vi "Test Encode to File Buffer.vi"(8 "error in (no error)":errorcluster, 11 "01_Image in":refnum<class "01_Image.lvclass">) -> (0 "error out":errorcluster, 3 "01_Image out":refnum<class "01_Image.lvclass">)   [LabVIEW 2020, in "test.lvlib" / "01_Image.lvclass"]
uses:
  01_Image.lvclass
  C:/Program Files (x86)/National Instruments/LabVIEW 2020/vi.lib/Astemes/LUnit/Test Case.lvclass
  common/Image Size (Integer).ctl
  <vilib>/Astemes/LUnit/Test Case.lvclass/Test Case.ctl
  image/Image to File-Buffer Encoder/Image to File-Buffer Encoder.lvclass/Image to File-Buffer Encoder.ctl
  21d28007-5dca-4d87-b59f-e9153fb71e50.vi
  image/Image to File-Buffer Encoder/Encode Image (ARGB).vi
  fadc1fe5-6c10-4d26-80da-2e71b1445ac9.vi
  image/New Image.vi
  image/New Image (ARGB Preallocated).vi
  image/Copy Array to Image.vi
  image/Copy Array to Image (ARGB).vi
  image/Encode Image to File Buffer (ARGB).vi/b711c62e-7e14-408f-bb3b-a3086b0dc120.vi
  <vilib>/Astemes/LUnit/Core/LUnit Test Case/Private/Append Pass Result.vi
  <vilib>/Astemes/LUnit/Core/LUnit Test Case/Private/Append Fail Result.vi
  21d28007-5dca-4d87-b59f-e9153fb71e50.vi/9c5d11cd-9439-4240-a1ee-d9baace9c924.vi
  image/Image to File-Buffer Encoder/Encode Image (ARGB).vi/c8136873-c742-4257-b221-98e07a73ef51.vi
  fadc1fe5-6c10-4d26-80da-2e71b1445ac9.vi/9c5d11cd-9439-4240-a1ee-d9baace9c924.vi
  image/New Image (ARGB Preallocated).vi/3321fa97-f432-4e1e-8db9-a0df79aed21b.vi
  image/ARGB Colour to U32 Pixel Value.vi
  <vilib>/Astemes/LUnit/Core/LUnit Test Case/Private/Run In UI.vi
  <vilib>/Utility/error.llb/Clear Errors.vi
  <vilib>/Utility/error.llb/Error Cluster From Error Code.vi
  <vilib>/picture/pixmap.llb/Flatten Pixmap.vi
  image/Image to File-Buffer Encoder/Create (with Extension).vi
  common/common.lvlib
  image/image.lvlib
  image/Image to File-Buffer Encoder/Image to File-Buffer Encoder.lvclass
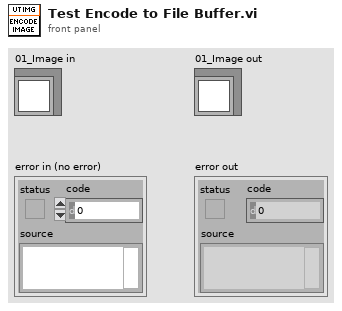
[diagram p1: front panel]
types:
  T1 = typedef "common.lvlib/Image Size (Integer).ctl" = cluster{"Width":u16, "Height":u16}
  T2 = typedef "image.lvlib/ARGB Image.ctl" = refnum<data-value>
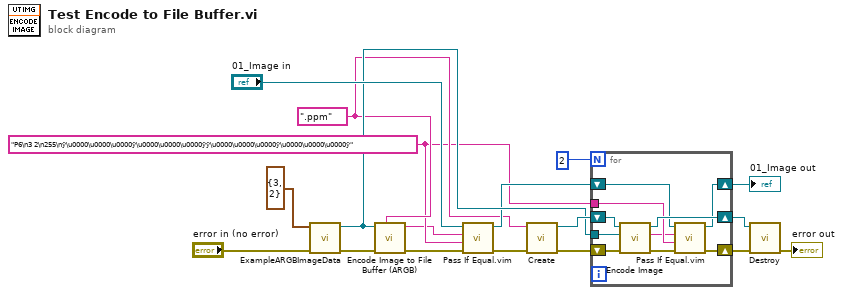
[diagram p0: block diagram]
diagram:
  w2 = "P6\n3 2\n255\nÿ\u0000\u0000\u0000ÿ\u0000\u0000\u0000ÿÿ\u0000\u0000\u0000ÿ\u0000\u0000\u0000ÿ" ("Buffer")
  w3 = ".ppm" ("Image File Extension")
  n1 = call "ExampleARGBImageData.vi"("error in (no error)"="error in (no error)", "Image Size"=T1 {"Width"=3, "Height"=2}) -> ("error out"=w16:errorcluster, "Data Value Reference out"=w12:T2)  [unwired: 6 in, 2 out]
  n2 = call "Encode Image to File Buffer (ARGB).vi"("Image File Extension"=w3, "error in (no error)"=w16, "ARGB Image Source in"=w12) -> ("error out"=w6:errorcluster, "Buffer"=w1:string)  [unwired: 7 in]
  n3 = call "Pass If Equal.vim"("error in (no error)"=w6, "Actual"=w2, "Expected"=w1, "LUnit Test Case In"="01_Image in") -> ("error out"=w5:errorcluster, "LUnit Test Case Out"=w8:refnum<class "01_Image.lvclass">)  [unwired: 6 in]
  n4 = call-poly "Create.vi"("error in (no error)"=w5, "Image File Extension"=w3) -> ("error out"=w11:errorcluster, "Image to File-Buffer Encoder"=w14:refnum<class "Image to File-Buffer Encoder.lvclass">)  [unwired: 8 in]
  n5 = for {
    N: 2 -> [_]
    shift-right: [w27] -> w9
    shift-left: w14 -> [w28]
    tunnel: w12 -> [w26]
    shift-right: [w21] -> w10
    shift-left: w11 -> [w25]
    shift-right: [w23] -> w7
    shift-left: w8 -> [w24]
    tunnel: w2 -> [w20]
    n6 = call-poly "Encode Image.vi"("error in (no error)"=w25, "ARGB Image"=w26, "Image to File-Buffer Encoder in"=w28) -> ("error out"=w22:errorcluster, "Buffer"=w19:string, "Image to File-Buffer Encoder"=w27:refnum<class "Image to File-Buffer Encoder.lvclass">)  [unwired: 6 in]
    n7 = call "Pass If Equal.vim"("error in (no error)"=w22, "Actual"=w20, "Expected"=w19, "LUnit Test Case In"=w24) -> ("error out"=w21:errorcluster, "LUnit Test Case Out"=w23:refnum<class "01_Image.lvclass">)  [unwired: 6 in]
  }
  "01_Image out" <- w7
  n8 = call "Destroy.vi"("error in (no error)"=w10, "Image to File-Buffer Encoder in"=w9) -> ("error out"=→"error out":errorcluster)  [unwired: 9 in]
